vi "Excel - Create And Save Docuement Tests.vi"(8 "error in (no error)":errorcluster) -> (0 "error out":errorcluster)   [LabVIEW 2017]
uses:
  src/LabVIEW NPOI/MS-Excel/MS-Excel.lvclass
  C:/Users/Neo/Desktop/Dev_Tools_BR/LabVIEW_NPOI/src/LabVIEW NPOI/Document/Document.lvclass
  src/LabVIEW NPOI/MS-Excel/Get Workbook.vi
  <vilib>/addons/_JKI Toolkits/Caraya/classes/Assert/Assert Not Error.vi
  <vilib>/addons/_JKI Toolkits/Caraya/classes/Assert/Assert False.vi
  <vilib>/addons/_JKI Toolkits/Caraya/classes/Assert/Assert True.vi
  C:/Users/Neo/Desktop/Dev_Tools_BR/LabVIEW_NPOI/lib/NPOI 2.1.1/NPOI.dll
  lib/NPOI 2.1.1/NPOI.dll
  src/LabVIEW NPOI/Document/Document.lvclass
  <vilib>/addons/_JKI Toolkits/Caraya/classes/Test/Test.lvclass
  <vilib>/addons/_JKI Toolkits/Caraya/classes/Assert/Assert.lvclass
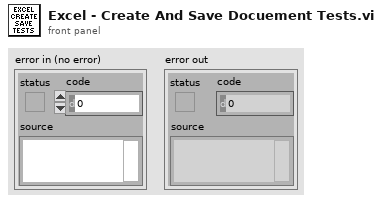
[diagram p1: front panel]
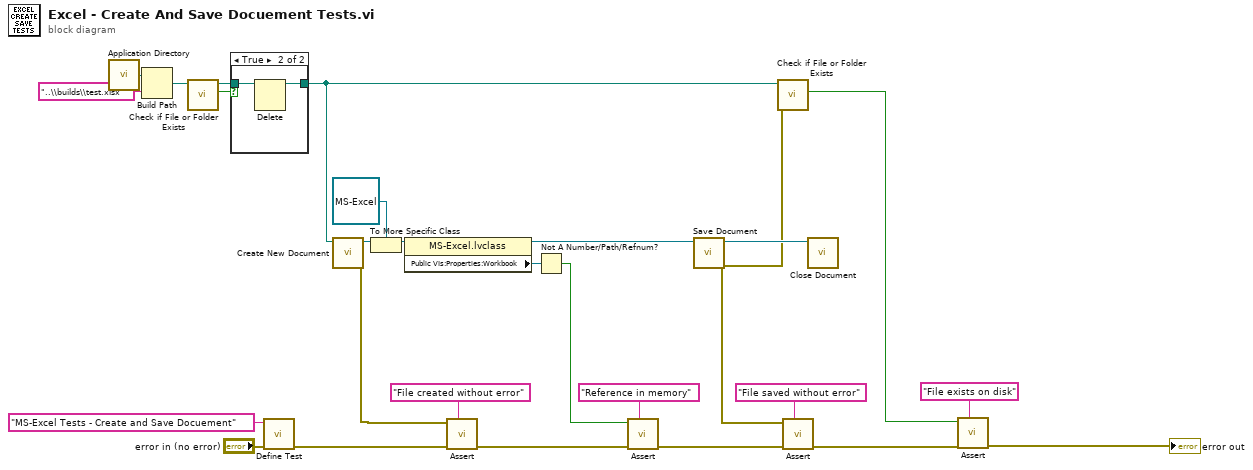
[diagram p0: block diagram]
diagram:
  n1 = call <vilib>:"Application Directory.vi"() -> ("Application Directory"=w6:path)
  n2 = Build Path(base path=w6, name or relative path="..\\builds\\test.xlsx" ("string")) -> (appended path=w4:path)
  n3 = call <vilib>:"Check if File or Folder Exists.vi"("path"=w4) -> ("file or folder exists?"=w16:bool, "dup path"=w15:path)  [unwired: 8 in, 1 out]
  n4 = case shown="True" w16 {
    tunnel: w15 -> [w28 w30]
    tunnel: [w28 w29] -> w3
    frame False {
    }
    frame True {
      n5 = Delete(path (use dialog)=w30) -> (deleted path=w29:path)  [unwired: 4 in, 2 out]
    }
  }
  n6 = call <vilib>:"Define Test.vi"("error in (no error)"="error in (no error)", "Label (VI Title)"="MS-Excel Tests - Create and Save Docuement") -> ("error out"=w26:errorcluster)  [unwired: 9 in]
  n7 = call "Create New Document.vi"("File Path"=w3) -> ("error out"=w24:errorcluster, "Document out"=w27:refnum<class "Document.lvclass">)  [unwired: 9 in]
  n8 = To More Specific Class(target class=refnum<class "MS-Excel.lvclass"> refnum ("LabVIEW NPOI.lvlib:MS-Excel.lvclass"), reference=w27) -> (specific class reference=w2:refnum<class "MS-Excel.lvclass">)  [unwired: 1 in, 1 out]
  n9 = property class="MS-Excel.lvclass"(reference=w2) -> (reference out=w18:refnum<class "MS-Excel.lvclass">, "Public VIs:Properties:Workbook"=w7:refnum<k24>)  [unwired: 1 in, 1 out]
  n10 = call-poly <vilib>:"Assert.vi"("Label"="File created without error", "error in (no error)"=w26, "Not Error?"=w24) -> ("error out"=w22:errorcluster)  [unwired: 8 in]
  n11 = Not A Number/Path/Refnum?(number/path/refnum=w7) -> (NaN/Path/Refnum?=w23:bool)
  n12 = call-poly <vilib>:"Assert.vi"("Label"="Reference in memory", "error in (no error)"=w22, "False?"=w23) -> ("error out"=w13:errorcluster)  [unwired: 8 in]
  n13 = call "Save Document.vi"("Document in"=w18) -> ("error out"=w9:errorcluster, "Document out"=w17:refnum<class "MS-Excel.lvclass">)  [unwired: 9 in]
  n14 = call <vilib>:"Check if File or Folder Exists.vi"("error in (no error)"=w9, "path"=w3) -> ("file or folder exists?"=w8:bool)  [unwired: 7 in, 2 out]
  n15 = call-poly <vilib>:"Assert.vi"("Label"="File saved without error", "error in (no error)"=w13, "Not Error?"=w9) -> ("error out"=w12:errorcluster)  [unwired: 8 in]
  n16 = call "Close Document.vi"("Document in"=w17) -> ()  [unwired: 10 in, 1 out]
  n17 = call-poly <vilib>:"Assert.vi"("Label"="File exists on disk", "error in (no error)"=w12, "True?"=w8) -> ("error out"=→"error out":errorcluster)  [unwired: 8 in]
